vi "Editor Context.vi"() -> (2 "Editor Context":refnum<vi>)   [LabVIEW 2020, in "Conditum-Tools.lvlib" / "Entity Editor.lvclass"]
uses:
  Entity Editor.lvclass
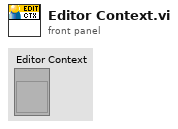
[diagram p1: front panel]
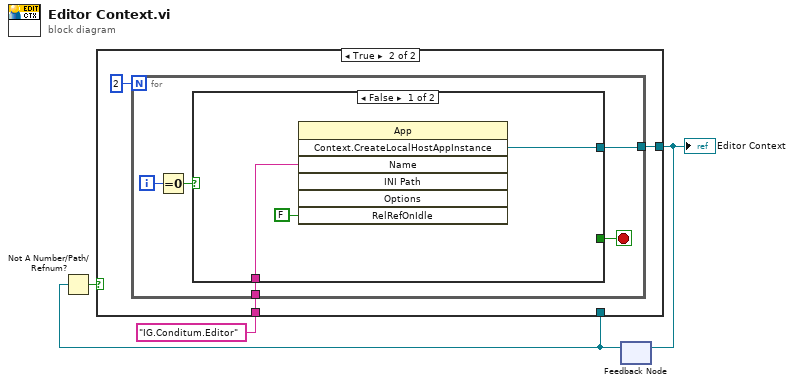
[diagram p0: block diagram]
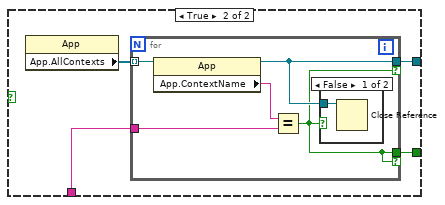
[diagram p3: hidden frame]
diagram:
  n1 = feedback #1() -> (w1:refnum<vi>)  [unwired: 1 in]
  n2 = Not A Number/Path/Refnum?(number/path/refnum=w1) -> (NaN/Path/Refnum?=w2:bool)
  n3 = case shown="True" w2 {
    tunnel: "IG.Conditum.Editor" -> [_ w7]
    tunnel: [w5 w6] -> w3
    tunnel: w1 -> [w5 _]
    frame False {
    }
    frame True {
      n4 = for {
        N: 2 -> [_]
        tunnel: w7 -> [w11]
        tunnel: [w9] -> w6
        i -> [w13]
        stop <- w10 stop-if-true
        n5 = Equal To 0?(x=w13) -> (x = 0?=w12:bool)
        n6 = case shown="False" w12 {
          tunnel: w11 -> [w15 w20]
          tunnel: [_ w18] -> w10
          tunnel: [w16 w17] -> w9
          frame False {
            n7 = invoke class="App" method="Context.CreateLocalHostAppInstance"("Name"=w15, "RelRefOnIdle"=FALSE ("Release Ref on Idle (T)")) -> ("Create Context"=w16:refnum<vi>)  [unwired: 5 in, 6 out]
          }
          frame True {
            n8 = property class="App"() -> ("App.AllContexts"=w19:refnum<vi>[])  [unwired: 2 in, 2 out]
            n9 = for {
              tunnel: w20 -> [w24]
              tunnel: w19 -> [w25] mode=indexing
              tunnel: [w22] -> w17 if=w21
              tunnel: [w21] -> w18 if=w21
              n10 = property class="App"(reference=w25) -> (reference out=w22:refnum<vi>, "App.ContextName"=w23:string)  [unwired: 1 in, 1 out]
              n11 = Equal?(x=w23, y=w24) -> (x = y?=w21:bool)
              n12 = case shown="False" w21 {
                tunnel: w22 -> [w26 _]
                frame False {
                  n13 = Close Reference(reference=w26) -> ()  [unwired: 1 in, 1 out]
                }
                frame True {
                }
              }
            }
          }
        }
      }
    }
  }
  "Editor Context" <- w3
  n14 = feedback-in #1(w3) -> ()
